vi "Create XLSX.vi"(7 "sheetname":string="Sheet1", 8 "error in (no error)":errorcluster, 10 "File Name":path) -> (0 "error out":errorcluster)   [LabVIEW 2013]
uses:
  C:/PhaeronGit/LVNPOI/Resources/NPOI 2.1.1 dotnet4/NPOI.OOXML.dll
  Resources/NPOI 2.1.1 dotnet4/NPOI.OOXML.dll
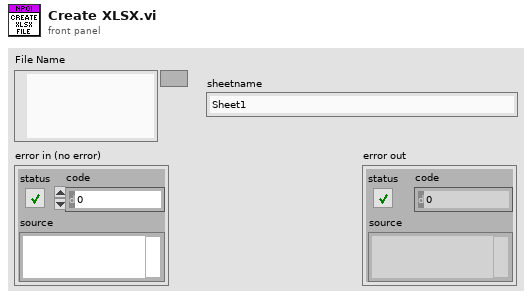
[diagram p1: front panel]
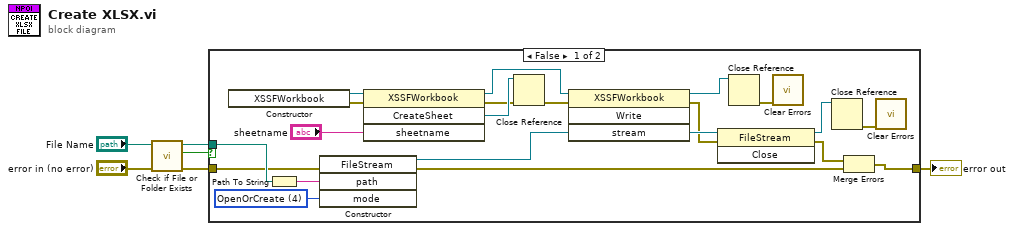
[diagram p0: block diagram]
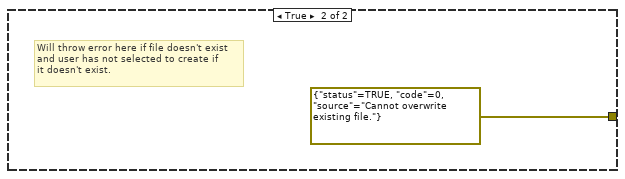
[diagram p2: hidden frame]
diagram:
  n1 = call <vilib>:"Check if File or Folder Exists.vi"("error in (no error)"="error in (no error)", "path"="File Name") -> ("error out"=w2:errorcluster, "file or folder exists?"=w1:bool, "dup path"=w3:path)  [unwired: 7 in]
  n2 = case shown="False" w1 {
    tunnel: [w21 errorcluster {"status"=TRUE, "code"=0, "source"="Cannot overwrite existing file."} ("error IO")] -> w6
    tunnel: w2 -> [w22 _]
    tunnel: w3 -> [w24 _]
    frame False {
      w26 = 4 items=["CreateNew"=1, "Create"=2, "Open"=3, "OpenOrCreate"=4, "Truncate"=5, "Append"=6] ("mode")
      n3 = constructor class="XSSFWorkbook"() -> (reference out=w16:refnum<k24>, error out=w15:errorcluster)  [unwired: 3 in, 1 out]
      n4 = Path To String(path=w24) -> (string=w25:string)
      n5 = constructor class="FileStream"(error in=w22, "path"=w25, "mode"=w26) -> (reference out=w11:refnum<k24>, error out=w19:errorcluster)  [unwired: 2 in, 3 out]
      n6 = invoke class="XSSFWorkbook" method="CreateSheet"(reference=w16, error in=w15, "sheetname"="sheetname") -> (reference out=w14:refnum<k24>, error out=w17:errorcluster, "CreateSheet"=w18:refnum<k24>)  [unwired: 1 in, 1 out]
      n7 = Close Reference(reference=w18, error in (no error)=w17) -> (error out=w13:errorcluster)
      n8 = invoke class="XSSFWorkbook" method="Write"(reference=w14, error in=w13, "stream"=w11) -> (reference out=w23:refnum<k24>, error out=w10:errorcluster)  [unwired: 1 in, 2 out]
      n9 = invoke class="FileStream" method="Close"(reference=w11, error in=w10) -> (reference out=w7:refnum<k24>, error out=w9:errorcluster)  [unwired: 1 in, 1 out]
      n10 = Close Reference(reference=w23) -> (error out=w20:errorcluster)  [unwired: 1 in]
      n11 = call <vilib>:"Clear Errors.vi"("error in (no error)"=w20) -> ()  [unwired: 6 in, 1 out]
      n12 = Close Reference(reference=w7) -> (error out=w8:errorcluster)  [unwired: 1 in]
      n13 = Merge Errors(w9, w19) -> (w21:errorcluster)
      n14 = call <vilib>:"Clear Errors.vi"("error in (no error)"=w8) -> ()  [unwired: 6 in, 1 out]
    }
    frame True {
      # "Will throw error here if file doesn't exist\nand user has not selected to create if\nit doesn't exist."
    }
  }
  "error out" <- w6
